vi "Sharp (SubVI).vi"(8 "error in (no error)":errorcluster) -> (0 "error out":errorcluster)   [LabVIEW 2017]
uses:
  <vilib>/myRIO/Instrument Drivers/Onboard IO/AI/vis/Read.vi
  <vilib>/myRIO/Instrument Drivers/Onboard IO/AI/vis/Smart Open.vi
  <vilib>/Utility/error.llb/Error Cluster From Error Code.vi
  <vilib>/myRIO/Common/Instrument Driver Framework/myRIO v1.0/AI/vis/myRIO v1.0 Read AI.vi
  Projects/Auto control/Inputs.vi
  <vilib>/ptbypt/NI_PtbyPt.lvlib
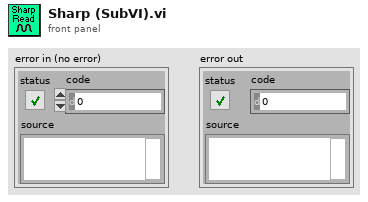
[diagram p1: front panel]
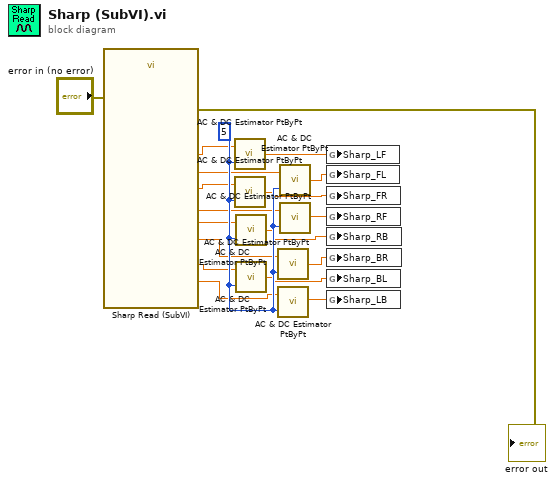
[diagram p0: block diagram]
diagram:
  w19 = 5 ("sample length")
  n1 = call "Sharp Read (SubVI).vi"("error in (no error)"="error in (no error)") -> ("BL (B/AI2 (Pin 7))"=w6:dbl, "LB (B/AI3 (Pin 9))"=w7:dbl, "LF (A/AI0 (Pin 3))"=w3:dbl, "FL (A/AI1 (Pin 5))"=w10:dbl, "FR (A/AI2 (Pin 7))"=w4:dbl, "RF (C/AI0 (AI0))"=w9:dbl, "RB (B/AI0 (Pin 3))"=w5:dbl, "BR (B/AI1 (Pin 5))"=w8:dbl, "error out"=→"error out":errorcluster)  [unwired: 18 in]
  n2 = call <vilib>:"AC & DC Estimator PtByPt.vi"("signal"=w3, "sample length"=w19) -> ("DC estimate (V)"=w11:dbl)  [unwired: 1 in, 2 out]
  n3 = call <vilib>:"AC & DC Estimator PtByPt.vi"("signal"=w4, "sample length"=w19) -> ("DC estimate (V)"=w13:dbl)  [unwired: 1 in, 2 out]
  n4 = call <vilib>:"AC & DC Estimator PtByPt.vi"("signal"=w5, "sample length"=w19) -> ("DC estimate (V)"=w15:dbl)  [unwired: 1 in, 2 out]
  n5 = call <vilib>:"AC & DC Estimator PtByPt.vi"("signal"=w6, "sample length"=w19) -> ("DC estimate (V)"=w17:dbl)  [unwired: 1 in, 2 out]
  n6 = call <vilib>:"AC & DC Estimator PtByPt.vi"("signal"=w8, "sample length"=w19) -> ("DC estimate (V)"=w16:dbl)  [unwired: 1 in, 2 out]
  n7 = call <vilib>:"AC & DC Estimator PtByPt.vi"("signal"=w7, "sample length"=w19) -> ("DC estimate (V)"=w18:dbl)  [unwired: 1 in, 2 out]
  n8 = call <vilib>:"AC & DC Estimator PtByPt.vi"("signal"=w10, "sample length"=w19) -> ("DC estimate (V)"=w12:dbl)  [unwired: 1 in, 2 out]
  n9 = call <vilib>:"AC & DC Estimator PtByPt.vi"("signal"=w9, "sample length"=w19) -> ("DC estimate (V)"=w14:dbl)  [unwired: 1 in, 2 out]
  n10 = global write "Inputs.vi" "Sharp_LF"(w11) -> ()
  n11 = global write "Inputs.vi" "Sharp_FL"(w12) -> ()
  n12 = global write "Inputs.vi" "Sharp_FR"(w13) -> ()
  n13 = global write "Inputs.vi" "Sharp_RF"(w14) -> ()
  n14 = global write "Inputs.vi" "Sharp_RB"(w15) -> ()
  n15 = global write "Inputs.vi" "Sharp_BR"(w16) -> ()
  n16 = global write "Inputs.vi" "Sharp_BL"(w17) -> ()
  n17 = global write "Inputs.vi" "Sharp_LB"(w18) -> ()
